vi "giltch_damaged_detector.vi"(10 "D":ext[](array[numeric]), 11 "side points":dbl[][](array[numeric])) -> (0 "damaged coord":dbl[](array[numeric]), 1 "giltch_coord":dbl[](array[numeric]), 2 "D_damaged":ext, 3 "D_giltch":ext)   [LabVIEW 2017]
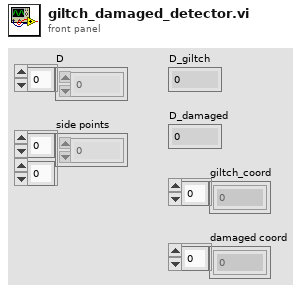
[diagram p1: front panel]
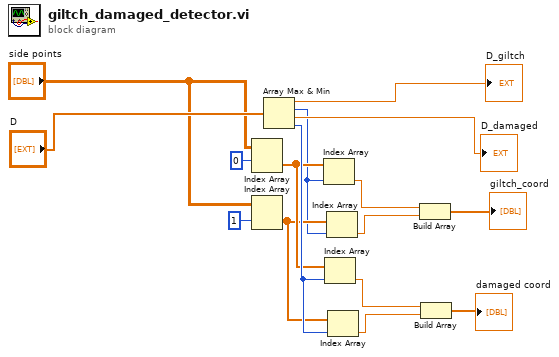
[diagram p0: block diagram]
diagram:
  n1 = Index Array(array="side points", index (row)=0) -> (element=w9:dbl[])  [unwired: 1 in]
  n2 = Index Array(array="side points", index (row)=1) -> (element=w8:dbl[])  [unwired: 1 in]
  n3 = Array Max & Min(array="D") -> (max value=→"D_giltch":ext, max index (indices)=w3:i32, min value=→"D_damaged":ext, min index (indices)=w10:i32)
  n4 = Index Array "Index Array"(array=w9, index=w3) -> (element=w4:dbl)
  n5 = Index Array(array=w9, index=w10) -> (element=w7:dbl)
  n6 = Index Array(array=w8, index=w3) -> (element=w5:dbl)
  n7 = Index Array(array=w8, index=w10) -> (element=w6:dbl)
  n8 = Build Array(w4, w5) -> (→"giltch_coord":dbl[])
  n9 = Build Array(w7, w6) -> (→"damaged coord":dbl[])
